vi "Get Scanner (Continuous).vi"(8 "error in (no error)":errorcluster, 11 "Power Supply in":refnum<class "Power Supply.lvclass">) -> (0 "error out":errorcluster, 2 "Continuous Scanner out":refnum<class "Continuous.lvclass">)   [LabVIEW 2009, in "Power Supply.lvclass"]
uses:
  Power Supply.lvclass
  Scanners/Magnetic Field/Continuous/Continuous.lvclass
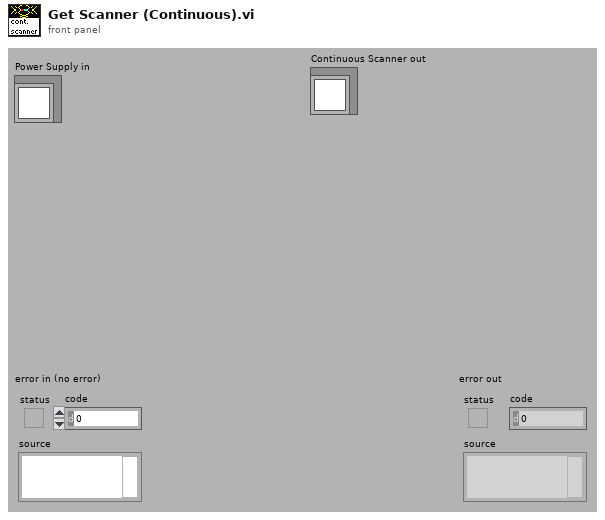
[diagram p1: front panel]
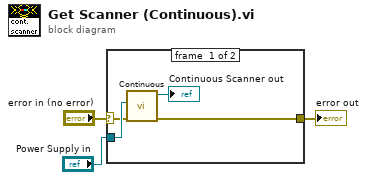
[diagram p0: block diagram]
diagram:
  n1 = case shown="No Error" "error in (no error)" {
    selector: "error in (no error)" -> [w5 w8]
    tunnel: [w4 w8] -> w2
    tunnel: "Power Supply in" -> [w7 _]
    frame #0 {
      n2 = call "Continuous.vi"("error in (no error)"=w5, "Power Supply in"=w7) -> ("error out"=w4:errorcluster, "Continuous.lvclass out"=→"Continuous Scanner out":refnum<class "Continuous.lvclass">)  [unwired: 8 out]
    }
    frame #1 {
    }
  }
  "error out" <- w2
